vi "Trigger.vi"(8 "error in (no error)":errorcluster, 11 "Reference in":T1={"Device"="GPIB0::4::INSTR", "Function"="", "delay"=20}) -> (0 "error out":errorcluster, 3 "Reference out":T1={"Device"="GPIB0::4::INSTR", "Function"="", "delay"=20}, 4 "question out":string)   [LabVIEW 2021, in "Rigol DM3052.lvlib"]
uses:
  Rigol DM3052.lvlib
  Reference.ctl
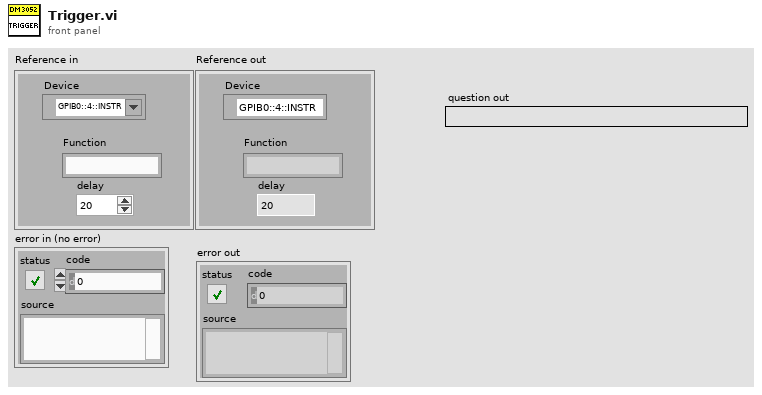
[diagram p1: front panel]
types:
  T1 = typedef "Rigol DM3052.lvlib/Reference.ctl" = cluster{"Device":refnum<visa-resource-name>, "Function":string, "delay":u32}
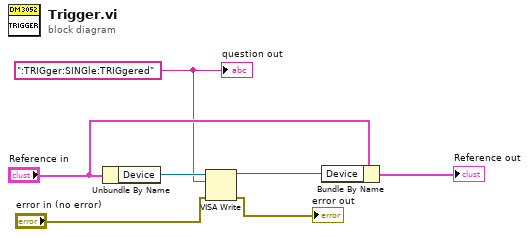
[diagram p0: block diagram]
diagram:
  w3 = ":TRIGger:SINGle:TRIGgered"
  n1 = Unbundle By Name("Reference in") -> ("Device"=w7:refnum<visa-resource-name>)
  n2 = VISA Write(VISA resource name=w7, write buffer=w3, error in (no error)="error in (no error)") -> (VISA resource name out=w5:refnum<visa-resource-name>, error out=→"error out":errorcluster)  [unwired: 1 out]
  n3 = Bundle By Name(cluster="Reference in", "Device"=w5) -> (→"Reference out":T1)
  "question out" <- w3
